vi "Get Config.vi"(8 "error in (no error)":errorcluster, 11 "Task in":refnum<class "Task.lvclass">) -> (0 "error out":errorcluster, 2 "Config":refnum<class "Task.lvclass">, 3 "Task out":refnum<class "Task.lvclass">)   [LabVIEW 2020, in "Volatus.lvlib" / "Task.lvclass"]
uses:
  Task.lvclass
  VolatusConfig/Task/Task.lvclass
  Task.lvclass/Task.ctl
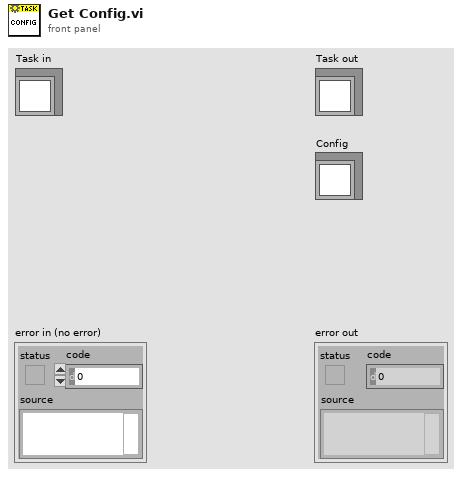
[diagram p1: front panel]
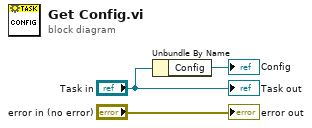
[diagram p0: block diagram]
diagram:
  n1 = Unbundle By Name("Task in") -> ("Config"=→"Config":refnum<class "Task.lvclass">)
  "error out" <- "error in (no error)"
  "Task out" <- "Task in"
